vi "Send Nested Value Update.vi"(7 "Message Priority (Normal)":T1=enum."Normal", 8 "Value":variant, 9 "Time (Get Time)":u32, 10 "Datum Name":string, 11 "Message Enqueuer":refnum<class "Message Enqueuer.lvclass">) -> (0 "error out":errorcluster, 3 "Message Enqueuer out":refnum<class "Message Enqueuer.lvclass">)   [LabVIEW 2017, in "IViewable.lvlib" / "Nested Value Update Msg.lvclass"]
doc: "This VI sends the message to an actor."
uses:
  Nested Value Update Msg.lvclass
  <vilib>/ActorFramework/Message Enqueuer/Message Enqueuer.lvclass
  <vilib>/ActorFramework/Message Enqueuer/Message Priority.ctl
  C:/Program Files (x86)/National Instruments/LabVIEW 2017/vi.lib/ActorFramework/Message/Message.lvclass
  Nested Value Update Msg.lvclass/Nested Value Update Msg.ctl
  <vilib>/ActorFramework/Message Enqueuer/Message Enqueuer.lvclass/Message Enqueuer.ctl
  <vilib>/ActorFramework/Message Priority Queue/Priority Enqueue.vi
panel:
  in  "error in (no error)":errorcluster
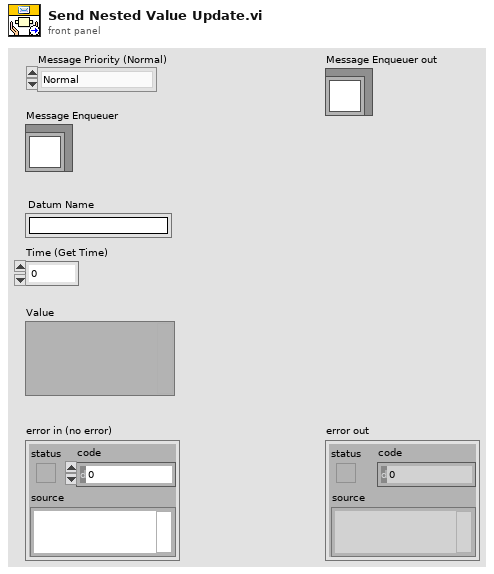
[diagram p1: front panel]
types:
  T1 = typedef "Actor Framework.lvlib/Message Enqueuer.lvclass/Message Priority.ctl" = enum16{"Low", "Normal", "High"}
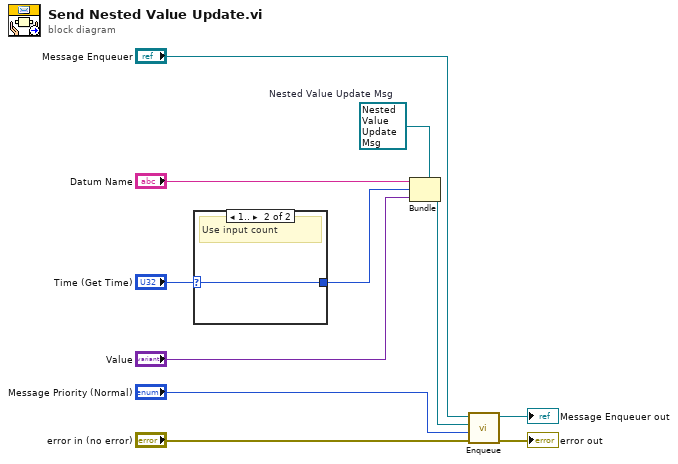
[diagram p0: block diagram]
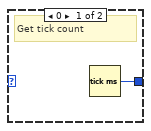
[diagram p2: hidden frame]
diagram:
  w6 = refnum<class "Nested Value Update Msg.lvclass"> refnum  # Nested Value Update Msg
  n1 = case shown="1.." "Time (Get Time)" {
    selector: "Time (Get Time)" -> [_ w13]
    tunnel: [w12 w13] -> w1
    frame 0 {
      # "Get tick count"
      n2 = Tick Count (ms)() -> (millisecond timer value=w12:u32)
    }
    frame 1.. {
      # "Use input count"
    }
  }
  n3 = Bundle(cluster=w6, "Datum Name", w1, "Value") -> (w5:refnum<class "Nested Value Update Msg.lvclass">)
  n4 = call <vilib>:"Enqueue.vi"("error in (no error)"="error in (no error)", "Message Priority (Normal)"="Message Priority (Normal)", "Message"=w5, "Message Enqueuer in"="Message Enqueuer") -> ("error out"=→"error out":errorcluster, "Message Enqueuer out"=→"Message Enqueuer out":refnum<class "Message Enqueuer.lvclass">)  [unwired: 6 in]
